vi "replace channel.vi"(8 "error in":errorcluster, 10 "channel":refnum<class "TBM channel.lvclass">, 11 "user module configuration in":refnum<class "fixed channel tag bus module configuration.lvclass">) -> (0 "error out":errorcluster, 3 "user module configuration out":refnum<class "fixed channel tag bus module configuration.lvclass">)   [LabVIEW 2013, in "fixed channel tag bus module configuration.lvclass"]
uses:
  fixed channel tag bus module configuration.lvclass
  <vilib>/NI/Tag Bus Module Framework/channel/TBM channel.lvclass
  fixed channel tag bus module configuration.lvclass/fixed channel tag bus module configuration.ctl
  <vilib>/NI/Tag Bus/tag/tag descriptor.lvclass/tag descriptor.ctl
  <vilib>/NI/Tag Bus/tag/read tag name.vi
  <vilib>/NI/Tag Bus/tag/tag descriptor.lvclass
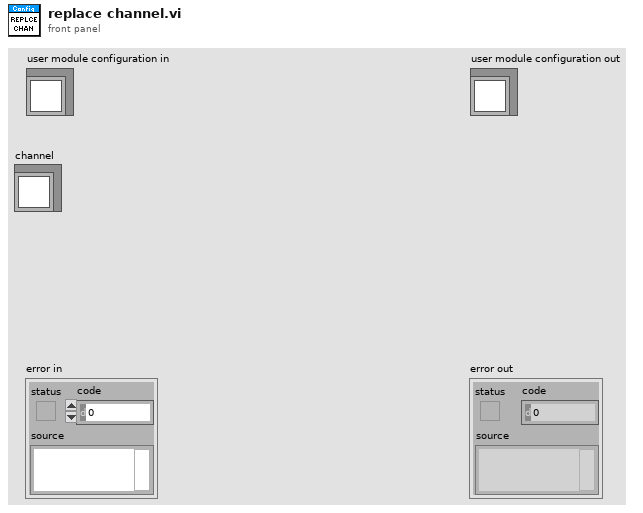
[diagram p1: front panel]
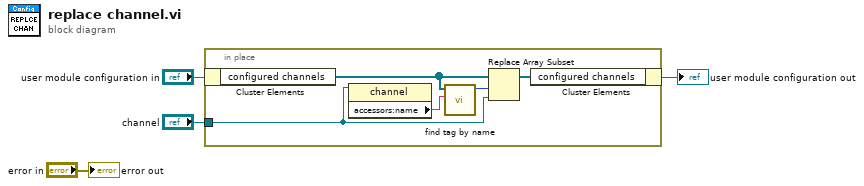
[diagram p0: block diagram]
diagram:
  n1 = in-place {
    in-place-border: "channel" -> [w6]
    n2 = in-place-cluster #1("user module configuration in") -> ("configured channels"=w9:refnum<class "TBM channel.lvclass">[])
    n3 = property class="channel"(reference=w6) -> ("accessors:name"=w5:string)  [unwired: 1 in, 2 out]
    n4 = call <vilib>:"find tag by name.vi"("name"=w5, "tags in"=w9) -> ("index"=w7:i32)  [unwired: 9 in]
    n5 = Replace Array Subset(array=w9, new element=w6, index=w7) -> (w8:refnum<class "TBM channel.lvclass">[])
    n6 = in-place-cluster #1("configured channels"=w8) -> (→"user module configuration out":refnum<class "fixed channel tag bus module configuration.lvclass">)
  }
  "error out" <- "error in"
